vi "ROI_Unbinned.vi"(6 "Scales IN":T4={"X Max"=1340.0, "Y Min"=1.0, "X Min"=1.0, "Y Max"=400.0}, 8 "CrsList":T2, 9 "Binning":u32=1, 10 "Use Cursors":bool, 11 "Parameters IN":T1={"camera parameters"={"Camera Handle"=16842752, "Xdim"=1340, "Ydim"=400}, "error"={"status"=FALSE, "code"=0, "source"=""}, "Plot height [pixel]"=1340.0, "Plot width [pixel]"=400.0}) -> (0 "Scales of Full Chip Plot":T4={"X Max"=1340.0, "Y Min"=1.0, "X Min"=1.0, "Y Max"=400.0}, 1 "Index 2":u32, 2 "Index 1":u32, 3 "Plot Area":T3, 4 "CrsList OUT":T2, 5 "ROI Parameters":T5, 7 "Parameters OUT":T1={"camera parameters"={"Camera Handle"=16842752, "Xdim"=1340, "Ydim"=400}, "error"={"status"=FALSE, "code"=0, "source"=""}, "Plot height [pixel]"=0.0, "Plot width [pixel]"=0.0})   [LabVIEW 2013]
uses:
  <vilib>/Utility/miscctls.llb/LVCursorListTypeDef.ctl
panel:
  in  "Eingang 3":T3
  out "Old Binning":u32=1
  in  "Eingang 1":T5
  # "Full Chip\nValues"
  # "1340"
  # "1"
  # "400"
  # "1"
  # "Full Chip\nValues"
  # "1340"
  # "1"
  # "400"
  # "1"
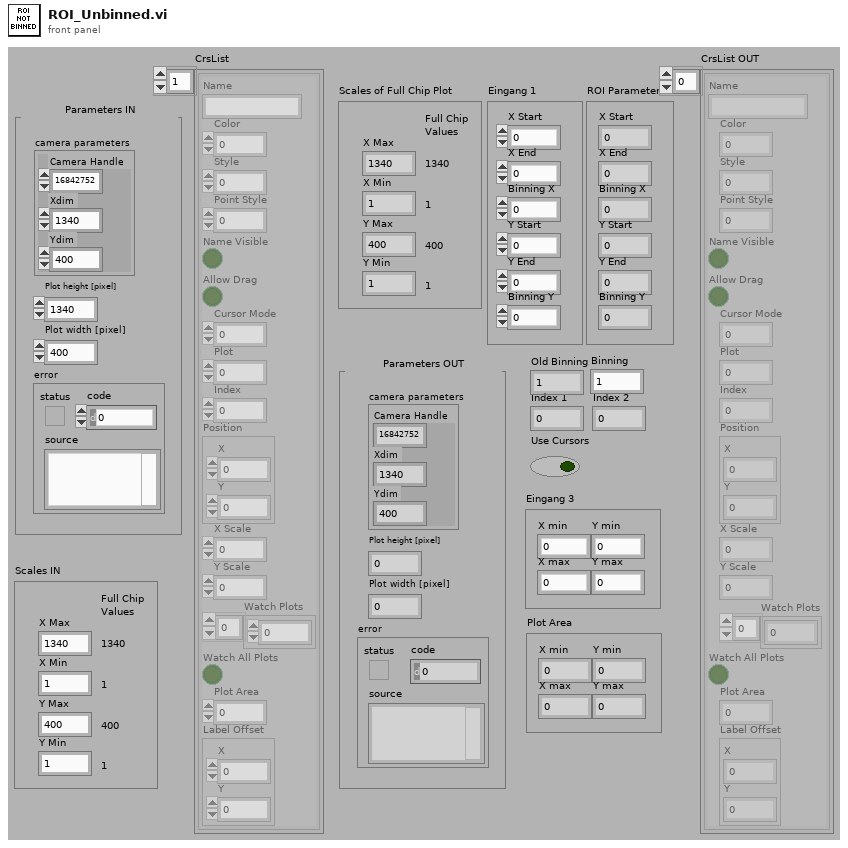
[diagram p1: front panel]
types:
  T1 = cluster{"camera parameters":cluster{"Camera Handle":u32, "Xdim":u32, "Ydim":u32}, "error":errorcluster, "Plot height [pixel]":dbl, "Plot width [pixel]":dbl}
  T2 = typedef "LVCursorListTypeDef.ctl" = cluster{"Name":string, "Color":u32, "Style":u8, "Point Style":u8, "Name Visible":bool, "Allow Drag":bool, "Cursor Mode":u32, "Plot":i32, "Index":i32, "Position":cluster{"X":dbl, "Y":dbl}, "X Scale":u32, "Y Scale":u32, "Watch Plots":i32[], "Watch All Plots":bool, "Plot Area":i32, "Label Offset":cluster{"X":dbl, "Y":dbl}}[]
  T3 = cluster{"X min":dbl, "Y min":dbl, "X max":dbl, "Y max":dbl}
  T4 = cluster{"X Max":dbl, "Y Min":dbl, "X Min":dbl, "Y Max":dbl}
  T5 = cluster{"X Start":u32, "X End":u32, "Binning X":u32, "Y Start":u32, "Y End":u32, "Binning Y":u32}
  T6 = cluster{"Name":string, "Color":u32, "Style":u8, "Point Style":u8, "Name Visible":bool, "Allow Drag":bool, "Cursor Mode":u32, "Plot":i32, "Index":i32, "Position":cluster{"X":dbl, "Y":dbl}, "X Scale":u32, "Y Scale":u32, "Watch Plots":i32[], "Watch All Plots":bool, "Plot Area":i32, "Label Offset":cluster{"X":dbl, "Y":dbl}}
  T7 = cluster{"Name":string, "Color":u32, "Style":u8, "Point Style":u8, "Name Visible":bool, "Allow Drag":bool, "Cursor Mode":u32, "Plot":i32, "Index":i32, "Position":cluster{"X":dbl, "Y":dbl}, "X Scale":u32, "Y Scale":u32, "Watch Plots":i32[], "Watch All Plots":bool, "Plot Area":i32, "Label Offset":cluster{"X":dbl, "Y":dbl}}[]
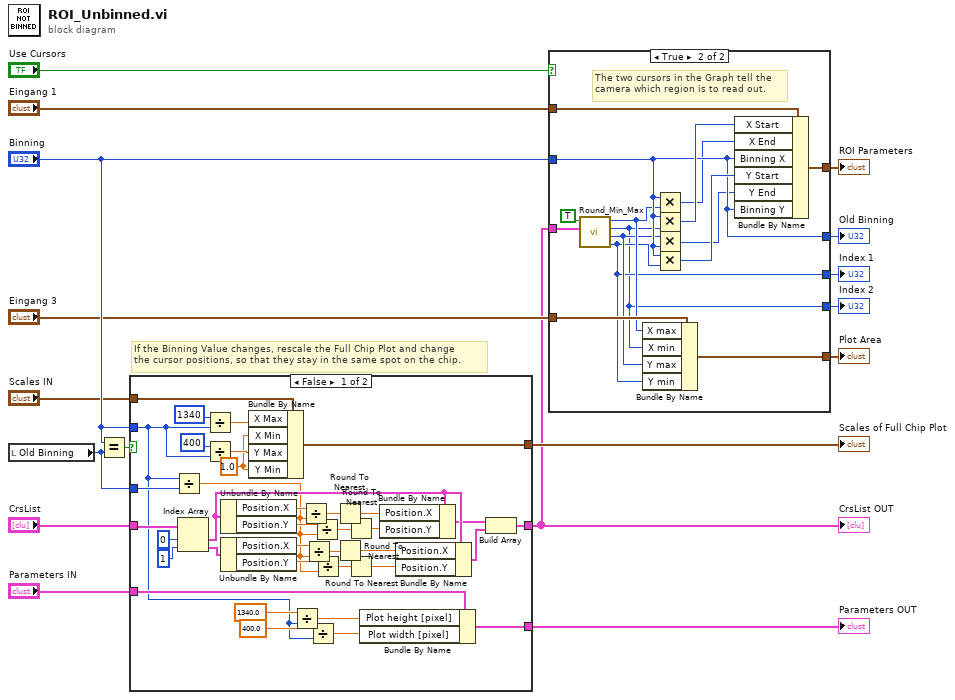
[diagram p0: block diagram]
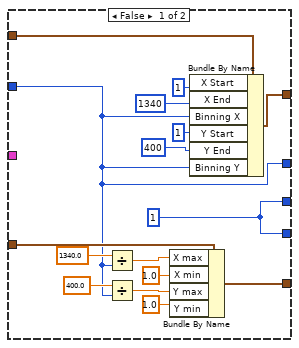
[diagram p3: hidden frame]
diagram:
  # "If the Binning Value changes, rescale the Full Chip Plot and change\nthe cursor positions, so that they stay in the same spot on the chip."
  n1 = local read "Old Binning"() -> (w4:u32)
  n2 = Equal?(x="Binning", y=w4) -> (x = y?=w6:bool)
  n3 = case shown="False" w6 {
    tunnel: [w53 w56] -> w7
    tunnel: "Binning" -> [w18 _]
    tunnel: "Scales IN" -> [w47 w56]
    tunnel: "CrsList" -> [w40 w55]
    tunnel: w4 -> [w39 _]
    tunnel: [w38 w55] -> w1
    tunnel: "Parameters IN" -> [w25 w54]
    tunnel: [w20 w54] -> w2
    frame False {
      w48 = 1.0 ("Y Min")
      n4 = Divide(x=w18, y=w39) -> (x/y=w19:dbl)
      n5 = Index Array(array=w40, index #1=0 ("index"), index #2=1 ("index")) -> (element #1=w43:T6, element #2=w44:T6)
      n6 = Divide(x=u32 1340, y=w18) -> (x/y=w50:dbl)
      n7 = Divide(x=u32 400, y=w18) -> (x/y=w49:dbl)
      n8 = Unbundle By Name(w43) -> ("Position.X"=w37:dbl, "Position.Y"=w36:dbl)
      n9 = Unbundle By Name(w44) -> ("Position.X"=w35:dbl, "Position.Y"=w34:dbl)
      n10 = Bundle By Name(cluster=w47, "X Max"=w50, "X Min"=w48, "Y Max"=w49, "Y Min"=w48) -> (w53:T4)
      n11 = Divide(x=1340.0, y=w18) -> (x/y=w22:dbl)
      n12 = Divide(x=w37, y=w19) -> (x/y=w33:dbl)
      n13 = Divide(x=w35, y=w19) -> (x/y=w31:dbl)
      n14 = Divide(x=400.0, y=w18) -> (x/y=w21:dbl)
      n15 = Divide(x=w36, y=w19) -> (x/y=w32:dbl)
      n16 = Divide(x=w34, y=w19) -> (x/y=w30:dbl)
      n17 = Round To Nearest(number=w33) -> (nearest integer value=w29:dbl)
      n18 = Round To Nearest(number=w31) -> (nearest integer value=w27:dbl)
      n19 = Round To Nearest(number=w32) -> (nearest integer value=w28:dbl)
      n20 = Round To Nearest(number=w30) -> (nearest integer value=w26:dbl)
      n21 = Bundle By Name(cluster=w25, "Plot height [pixel]"=w22, "Plot width [pixel]"=w21) -> (w20:T1)
      n22 = Bundle By Name(cluster=w43, "Position.X"=w29, "Position.Y"=w28) -> (w42:T6)
      n23 = Bundle By Name(cluster=w43, "Position.X"=w27, "Position.Y"=w26) -> (w41:T6)
      n24 = Build Array(w42, w41) -> (w38:T7)
    }
    frame True {
    }
  }
  "Scales of Full Chip Plot" <- w7
  "CrsList OUT" <- w1
  "Parameters OUT" <- w2
  n25 = case shown="True" "Use Cursors" {
    tunnel: "Eingang 1" -> [w68 w87]
    tunnel: [w67 w86] -> w16
    tunnel: [w66 w75] -> w15
    tunnel: [w66 w74] -> w14
    tunnel: w1 -> [_ w85]
    tunnel: "Binning" -> [w57 w82]
    tunnel: [w57 w82] -> w11
    tunnel: "Eingang 3" -> [w65 w80]
    tunnel: [w64 w77] -> w9
    frame False {
      w66 = u32 1 ("min(Y)")
      n26 = Divide(x=1340.0 ("X max"), y=w57) -> (x/y=w60:dbl)
      n27 = Divide(x=400.0 ("Y max"), y=w57) -> (x/y=w61:dbl)
      n28 = Bundle By Name(cluster=w65, "X max"=w60, "X min"=1.0, "Y max"=w61, "Y min"=1.0) -> (w64:T3)
      n29 = Bundle By Name(cluster=w68, "X Start"=u32 1, "X End"=u32 1340, "Binning X"=w57, "Y Start"=u32 1, "Y End"=u32 400, "Binning Y"=w57) -> (w67:T5)
    }
    frame True {
      # "The two cursors in the Graph tell the\ncamera which region is to read out."
      n30 = call "Round_Min_Max.vi"("CrsList"=w85, "Use Cursors"=TRUE) -> ("min(Y)"=w75:u32, "max(Y)"=w78:u32, "min(X)"=w74:u32, "max(X)"=w79:u32)  [unwired: 6 in]
      n31 = Bundle By Name(cluster=w80, "X max"=w79, "X min"=w74, "Y max"=w78, "Y min"=w75) -> (w77:T3)
      n32 = Multiply(x=w82, y=w79) -> (x*y=w76:u32)
      n33 = Multiply(x=w82, y=w74) -> (x*y=w84:u32)
      n34 = Multiply(x=w78, y=w82) -> (x*y=w81:u32)
      n35 = Multiply(x=w82, y=w75) -> (x*y=w83:u32)
      n36 = Bundle By Name(cluster=w87, "X Start"=w84, "X End"=w76, "Binning X"=w82, "Y Start"=w83, "Y End"=w81, "Binning Y"=w82) -> (w86:T5)
    }
  }
  "ROI Parameters" <- w16
  "Index 1" <- w15
  "Index 2" <- w14
  "Old Binning" <- w11
  "Plot Area" <- w9
